vi "S2DS_ComputeWCDirection.vi"(11 "Sweep info in":T1 {"Y data taking" items=["in both direction", "in up direction only", "in down direction only"]; "X data taking" items=["in both direction", "in up direction only", "in down direction only"]}) -> (1 "Change  x direction":bool, 2 "Change y direction":bool, 3 "Sweep info out":T1 {"Y data taking" items=["in both direction", "in up direction only", "in down direction only"]; "X data taking" items=["in both direction", "in up direction only", "in down direction only"]})   [LabVIEW 2016]
uses:
  TYPE DEFS/S2DS_Sweep Info.ctl
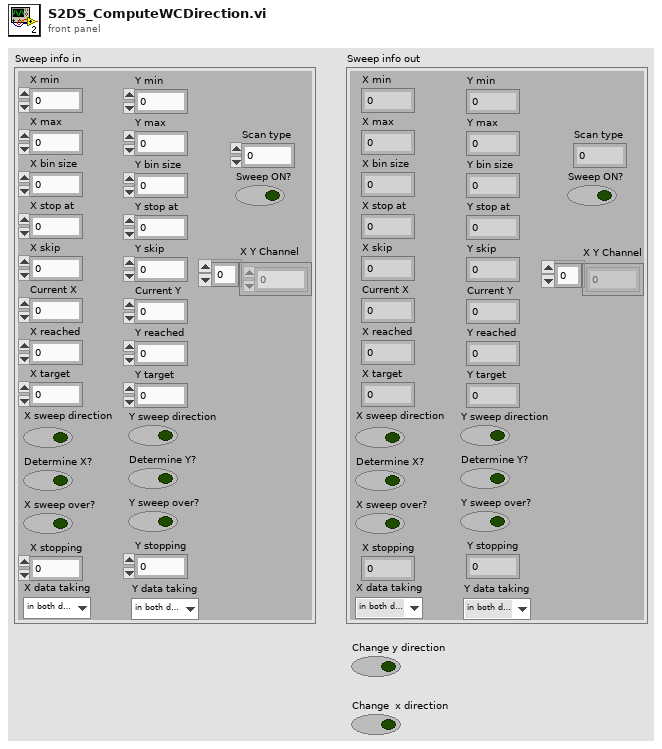
[diagram p1: front panel]
types:
  T1 = typedef "S2DS_Sweep Info.ctl" = cluster{"X min":ext, "X max":dbl, "Y min":dbl, "Y max":dbl, "X bin size":dbl, "Y bin size":dbl, "X stop at":dbl, "Y stop at":dbl, "X skip":u64, "Y skip":u64, "Current X":dbl, "Current Y":dbl, "X reached":i32, "Y reached":i32, "X target":dbl, "Y target":dbl, "Sweep ON?":bool, "X sweep direction":bool, "Y sweep direction":bool, "Determine X?":bool, "Determine Y?":bool, "X sweep over?":bool, "Y sweep over?":bool, "Scan type":i32, "X stopping":i32, "Y stopping":i32, "X Y Channel":u16[], "X data taking":u16, "Y data taking":u16}
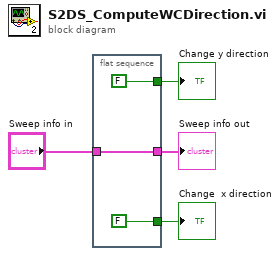
[diagram p0: block diagram]
diagram:
  n1 = flat-sequence {
    tunnel: "Sweep info in" -> [w7]
    tunnel: [w7] -> w2
    tunnel: [FALSE ("Change y direction")] -> w3
    tunnel: [FALSE ("Change  x direction")] -> w4
    frame #0 {
    }
  }
  "Change  x direction" <- w4
  "Change y direction" <- w3
  "Sweep info out" <- w2
